vi "best_angle.vi"(2 "Waypoint Heading":dbl, 3 "Current Heading":dbl, 4 "Wind Vector":cluster{"Wind R":dbl, "Wind Theta":dbl}) -> (1 "Best Angle":dbl)   [LabVIEW 2011]
panel:
  in  "thres+":dbl=2.0
  in  "thresh x":dbl=1.2
  out "Numeric":i32
  out "Angle2":dbl
  out "Angle1":dbl
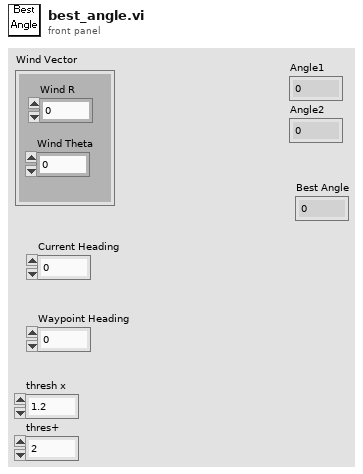
[diagram p1: front panel]
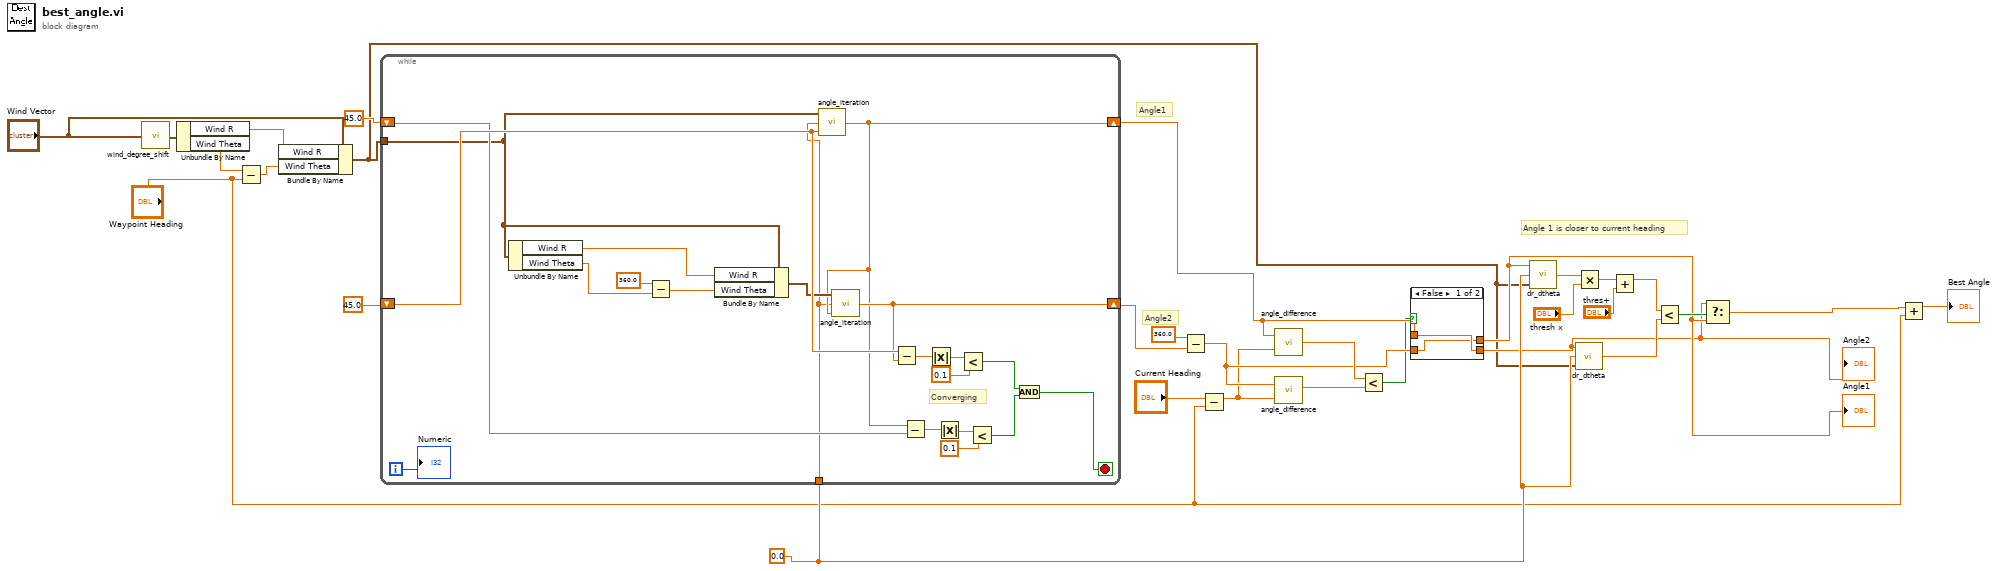
[diagram p0: block diagram]
diagram:
  w22 = 0.0
  # "Angle 1 is closer to current heading"
  # "Angle2"
  # "Angle1"
  n1 = call "wind_degree_shift.vi"("Wind Vector -180 - 180"="Wind Vector") -> ("Wind Vector 0-360"=w21:cluster{"Wind R":dbl, "Wind Theta":dbl})
  n2 = Unbundle By Name(w21) -> ("Wind R"=w20:dbl, "Wind Theta"=w18:dbl)
  n3 = Subtract(x=w18, y="Waypoint Heading") -> (x-y=w19:dbl)
  n4 = Bundle By Name(cluster="Wind Vector", "Wind R"=w20, "Wind Theta"=w19) -> (w3:cluster{"Wind R":dbl, "Wind Theta":dbl})
  n5 = while {
    shift-right: [w47] -> w26
    shift-left: 45.0 ("Best Theta") -> [w48]
    tunnel: w3 -> [w35]
    shift-right: [w32] -> w11
    shift-left: 45.0 ("Best Theta") -> [w43]
    tunnel: w22 -> [w31]
    i -> [w39]
    stop <- w40 stop-if-true
    # "Converging"
    n6 = Unbundle By Name(w35) -> ("Wind R"=w33:dbl, "Wind Theta"=w37:dbl)
    n7 = Subtract(x=360.0, y=w37) -> (x-y=w34:dbl)
    n8 = Bundle By Name(cluster=w35, "Wind R"=w33, "Wind Theta"=w34) -> (w36:cluster{"Wind R":dbl, "Wind Theta":dbl})
    n9 = call "angle_iteration.vi"("Phi"=w48, "Goal Angle"=w31, "Wind Vector"=w35) -> ("Best Theta"=w32:dbl)
    n10 = call "angle_iteration.vi"("Phi"=w32, "Goal Angle"=w31, "Wind Vector"=w36) -> ("Best Theta"=w47:dbl)
    n11 = Subtract(x=w48, y=w47) -> (x-y=w51:dbl)
    n12 = Subtract(x=w32, y=w43) -> (x-y=w44:dbl)
    n13 = Absolute Value(x=w51) -> (abs(x)=w50:dbl)
    n14 = Absolute Value(x=w44) -> (abs(x)=w45:dbl)
    n15 = Less?(x=w50, y=0.1) -> (x < y?=w42:bool)
    n16 = Less?(x=w45, y=0.1) -> (x < y?=w41:bool)
    n17 = And(x=w42, y=w41) -> (x .and. y?=w40:bool)
    "Numeric" <- w39
  }
  n18 = Subtract(x=360.0, y=w26) -> (x-y=w8:dbl)
  n19 = Subtract(x="Current Heading", y="Waypoint Heading") -> (x-y=w2:dbl)
  n20 = call "angle_difference.vi"("Angle 2"=w2, "Angle 1"=w11) -> ("Difference"=w24:dbl)
  n21 = call "angle_difference.vi"("Angle 2"=w2, "Angle 1"=w8) -> ("Difference"=w25:dbl)
  n22 = Less?(x=w24, y=w25) -> (x < y?=w7:bool)
  n23 = case shown="False" w7 {
    tunnel: w11 -> [w53 w55]
    tunnel: [w52 w55] -> w10
    tunnel: [w53 w54] -> w9
    tunnel: w8 -> [w52 w54]
    frame False {
    }
    frame True {
    }
  }
  "Angle1" <- w10
  "Angle2" <- w9
  n24 = call "dr_dtheta.vi"("Wind Vector"=w3, "Goal Angle"=w22, "Boat Angle"=w10) -> ("dr/dtheta"=w16:dbl)
  n25 = call "dr_dtheta.vi"("Wind Vector"=w3, "Goal Angle"=w22, "Boat Angle"=w9) -> ("dr/dtheta"=w13:dbl)
  n26 = Multiply(x=w16, y="thresh x") -> (x*y=w12:dbl)
  n27 = Add(x=w12, y="thres+") -> (x+y=w6:dbl)
  n28 = Less?(x=w6, y=w13) -> (x < y?=w14:bool)
  n29 = Select(t=w9, s=w14, f=w10) -> (s? t:f=w29:dbl)
  n30 = Add(x=w29, y="Waypoint Heading") -> (x+y=→"Best Angle":dbl)
